vi "NodMcu interlink labview_3.vi"() -> ()   [LabVIEW 2015]
panel:
  in  "Tab Control":enum32{"Page 1", "Page 2"}(tab)
  in  "Switch":bool
  out "Alert_Message":string
  in  "stop":bool
  in  "IP":string
  # "Pardeep kumar"
  # "Nodmcu data to labview wih \n     Adafruit.io Cloud(IOT)"
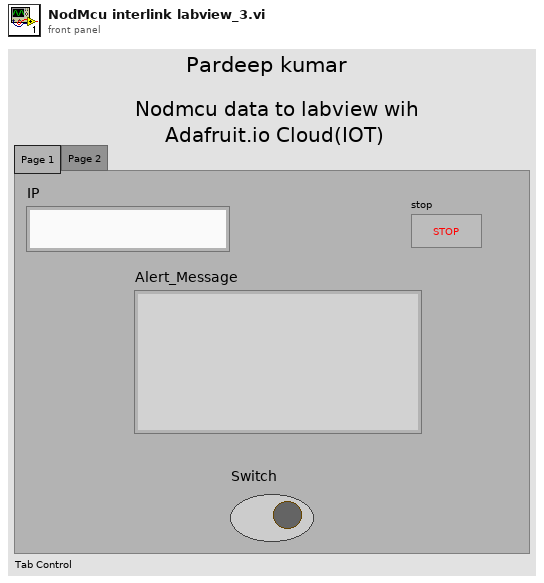
[diagram p1: front panel]
types:
  T1 = enum16{"Standard", "Buffered", "CRLF", "Immediate"}
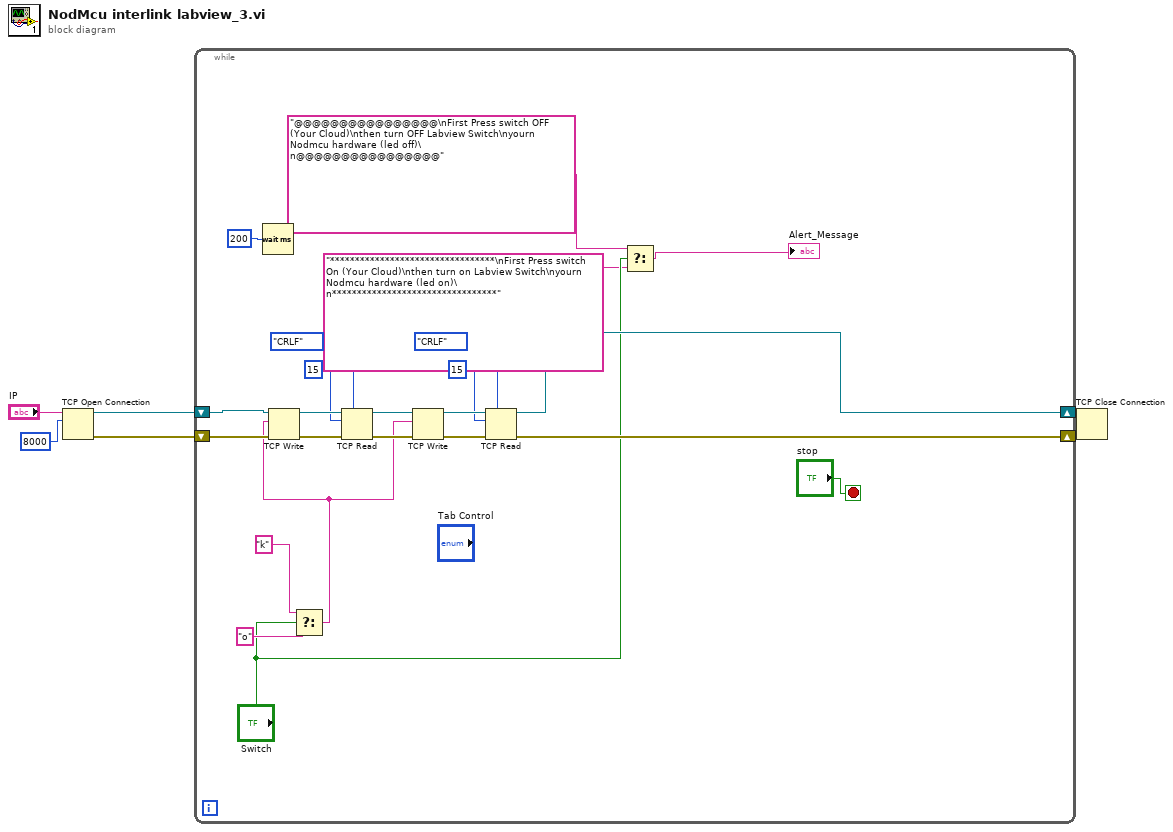
[diagram p0: block diagram]
diagram:
  n1 = TCP Open Connection(address="IP", remote port or service name=u16 8000) -> (connection ID=w4:refnum<k5>, error out=w3:errorcluster)  [unwired: 3 in]
  n2 = while {
    shift-right: [w19] -> w2
    shift-left: w4 -> [w29]
    shift-right: [w16] -> w1
    shift-left: w3 -> [w28]
    stop <- "stop" stop-if-true
    n3 = Wait (ms)(milliseconds to wait=u32 200) -> ()  [unwired: 1 out]
    n4 = Select(t="k", s="Switch", f="o" ("data in")) -> (s? t:f=w12:string)
    n5 = TCP Write(connection ID=w29, data in=w12, error in (no error)=w28) -> (connection ID out=w27:refnum<k5>, error out=w26:errorcluster)  [unwired: 1 in, 1 out]
    n6 = TCP Read(connection ID=w27, bytes to read=15, error in (no error)=w26, 7:T1."CRLF" ("mode (standard)")) -> (connection ID out=w21:refnum<k5>, error out=w18:errorcluster)  [unwired: 1 in, 1 out]
    n7 = TCP Write(connection ID=w21, data in=w12, error in (no error)=w18) -> (connection ID out=w20:refnum<k5>, error out=w17:errorcluster)  [unwired: 1 in, 1 out]
    n8 = TCP Read(connection ID=w20, bytes to read=15, error in (no error)=w17, 7:T1."CRLF" ("mode (standard)")) -> (connection ID out=w19:refnum<k5>, error out=w16:errorcluster)  [unwired: 1 in, 1 out]
    n9 = Select(t="@@@@@@@@@@@@@@@@\nFirst Press switch OFF (Your Cloud)\nthen turn OFF Labview Switch\nyourn Nodmcu hardware (led off)\n@@@@@@@@@@@@@@@@", s="Switch", f="*********************************\nFirst Press switch On (Your Cloud)\nthen turn on Labview Switch\nyourn Nodmcu hardware (led on)\n*********************************") -> (s? t:f=→"Alert_Message":string)
  }
  n10 = TCP Close Connection(connection ID=w2, error in (no error)=w1) -> ()  [unwired: 1 in, 2 out]
